vi "offset.vi"() -> ()   [LabVIEW 2020]
uses:
  bin/gepit.cp310.32.dll
panel:
  out "x-y":u64
  out "d":i32
  out "c":i32
  out "b":i32
  out "a":i32
  out "return type":i32
  out "sum":u8
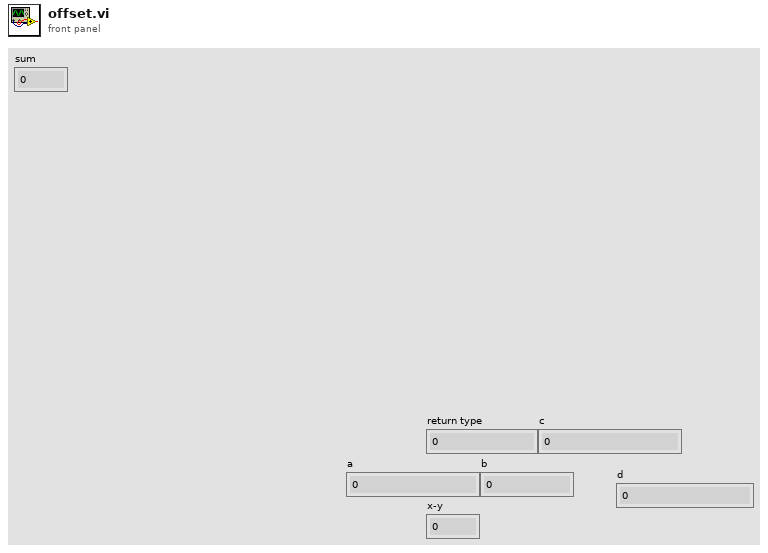
[diagram p1: front panel]
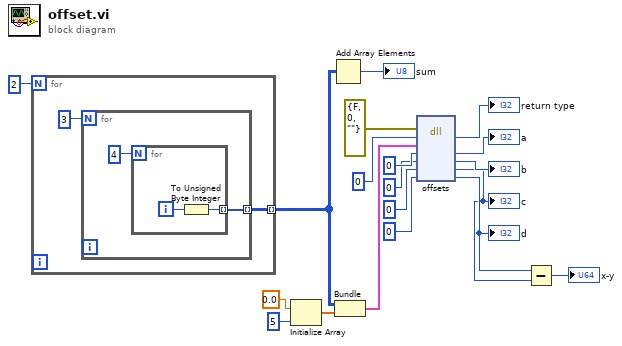
[diagram p0: block diagram]
diagram:
  n1 = for {
    N: 2 -> [_]
    tunnel: [w21] -> w15 mode=indexing
    n2 = for {
      N: 3 -> [_]
      tunnel: [w22] -> w21 mode=indexing
      n3 = for {
        N: 4 -> [_]
        tunnel: [w24] -> w22 mode=indexing
        i -> [w25]
        n4 = To Unsigned Byte Integer(number=w25) -> (unsigned 8bit integer=w24:u8)
      }
    }
  }
  n5 = Initialize Array(0.0, 5 ("dimension size")) -> (w14:dbl[])
  n6 = Add Array Elements(numeric array=w15) -> (sum=→"sum":u8)
  n7 = Bundle(w15, w14) -> (w13:cluster{u8[][][], dbl[]})  [unwired: 1 in]
  n8 = dll-call lib="C:/serenial/libraries/g-embedded-python-interpreter-toolkit/LabVIEW/bin/gepit.cp310.32.dll" fn="offsets"(error in=errorcluster {"status"=FALSE, "code"=0, "source"=""} ("error in (no error)"), "return type"=0, "arg2"=w13, "a"=0, "b"=0, "c"=0, "d"=0) -> ("return type"=→"return type":i32, "a"=→"a":u64, "b"=→"b":u64, "c"=w2:u64, "d"=w3:u64)  [unwired: 2 in, 2 out]
  "c" <- w2
  "d" <- w3
  n9 = Subtract(x=w3, y=w2) -> (x-y=→"x-y":u64)
